vi "格式化存.vi"() -> ()   [LabVIEW 2018]
panel:
  in  "数值":dbl
  in  "布尔":bool
  in  "字符串":string
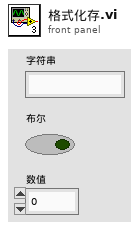
[diagram p1: front panel]
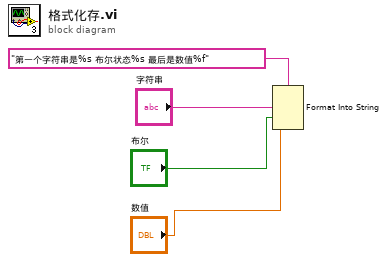
[diagram p0: block diagram]
diagram:
  n1 = Format Into String(format string="第一个字符串是%s 布尔状态%s 最后是数值%f" ("格式字符串"), "字符串", "布尔", "数值") -> ()  [unwired: 2 in, 2 out]
